vi "Definition Cluster.vi"(11 "Boolean in":refnum<class "Boolean.lvclass">) -> (2 "Definition":variant, 3 "Boolean out":refnum<class "Boolean.lvclass">)   [LabVIEW 2020, in "Conditum.lvlib" / "Columns.lvlib" / "Boolean.lvclass"]
uses:
  Boolean.lvclass
  Boolean.lvclass/Boolean.ctl
  Type/Definition.ctl
  Type/Type.lvclass
  Attributes.ctl
  Conditum.lvlib
  Definition.ctl
  Boolean Definition.ctl
  C:/dev/lv20CE/lv-conditum/Conditum/Columns/Type/Type.lvclass
  C:/dev/lv20CE/lv-conditum/Conditum/Columns/Boolean/Boolean.lvclass
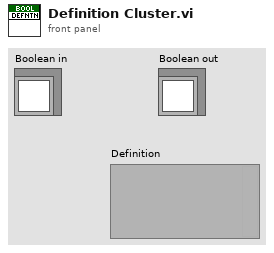
[diagram p1: front panel]
types:
  T1 = typedef "Conditum.lvlib/Columns.lvlib/Boolean.lvclass/Boolean Definition.ctl" = cluster{"Type":T2, "Attributes":T3, "Boolean":T4}
  T2 = typedef "Conditum.lvlib/Columns.lvlib/Type.lvclass/Definition.ctl" = cluster{"Name":string, "Nullable":bool, "Default NULL":bool}
  T3 = typedef "Conditum.lvlib/Attributes.ctl" = cluster{"Primary Key":bool, "Unique":bool, "Foreign Key":bool, "Auto Increment":bool}
  T4 = typedef "Conditum.lvlib/Columns.lvlib/Boolean.lvclass/Definition.ctl" = cluster{"Default":bool}
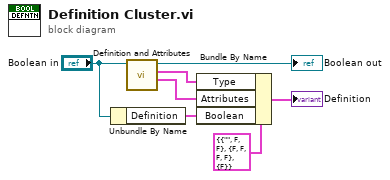
[diagram p0: block diagram]
diagram:
  n1 = Unbundle By Name("Boolean in") -> ("Definition"=w4:T4)
  n2 = call "Definition and Attributes.vi"("Type in"="Boolean in") -> ("Attributes"=w2:T3, "Definition"=w3:T2, "Type out"=→"Boolean out":refnum<class "Boolean.lvclass">)  [unwired: 8 in]
  n3 = Bundle By Name(cluster=T1 {"Type"={"Name"="", "Nullable"=FALSE, "Default NULL"=FALSE}, "Attributes"={"Primary Key"=FALSE, "Unique"=FALSE, "Foreign Key"=FALSE, "Auto Increment"=FALSE}, "Boolean"={"Default"=FALSE}} ("Definition"), "Type"=w3, "Attributes"=w2, "Boolean"=w4) -> (→"Definition":T1)
